vi "例5.2“数组大小”函数.vi"() -> ()   [LabVIEW 2017]
panel:
  out "大小":i32[](array[numeric])
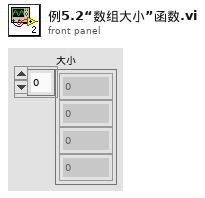
[diagram p1: front panel]
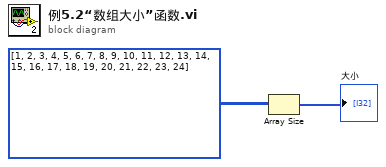
[diagram p0: block diagram]
diagram:
  n1 = Array Size(array=i32[][][] [[[1, 2, 3, 4], [5, 6, 7, 8], [9, 10, 11, 12]], [[13, 14, 15, 16], [17, 18, 19, 20], [21, 22, 23, 24]]]) -> (size(s)=→"大小":i32[])
